vi "Validate_Rect_Default.vi"(0 "rect":T1, 1 "default":T1) -> (2 "out":T1)   [LabVIEW 2012]
uses:
  <userlib>/BIAS2/subvis/ROI_rect.ctl
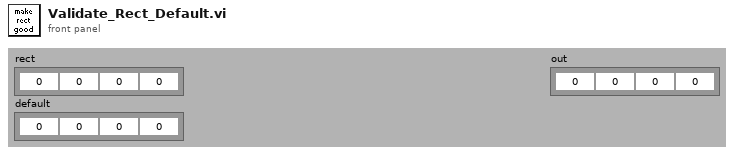
[diagram p1: front panel]
types:
  T1 = typedef "ROI_rect.ctl" = cluster{"left":i32, "top":i32, "right":i32, "bottom":i32}
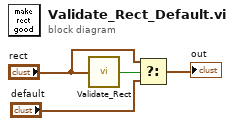
[diagram p0: block diagram]
diagram:
  n1 = call <userlib>:"Validate_Rect.vi"("rect"="rect") -> ("valid"=w4:bool)
  n2 = Select(t="rect", s=w4, f="default") -> (s? t:f=→"out":T1)
